vi "BinaryToFullScale.vi"(1 "Array 2":i16[](array[numeric])) -> (0 "Array":i16[](array[numeric]))   [LabVIEW 2014]
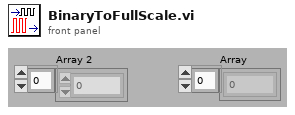
[diagram p1: front panel]
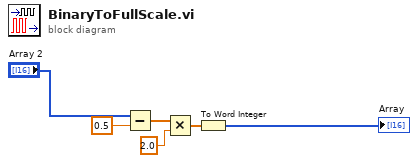
[diagram p0: block diagram]
diagram:
  n1 = Subtract(x="Array 2", y=0.5) -> (x-y=w3:dbl[])
  n2 = Multiply(x=w3, y=2.0) -> (x*y=w5:dbl[])
  n3 = To Word Integer(number=w5) -> (16bit integer=→"Array":i16[])
